vi "Actor Core.vi"(8 "error in":errorcluster, 11 "State in":refnum<class "Driver-Virtual.lvclass">) -> (0 "error out":errorcluster, 3 "Actor out":refnum<class "Actor.lvclass">)   [LabVIEW 2013, in "Virtual Systems.lvlib" / "Driver.lvlib" / "Driver-Virtual.lvclass"]
doc: "(<B>Filename</B>: Actor Framework.lvlib:Actor.lvclass:Actor Core.vi)\n\nThis override invokes Entry.vi on the initial state, prior to calling the parent Actor Core. Adding this behavior to Actor Core (instead of an override of Pre Launch Init.vi) allows the initial state to launch a nested actor as part of its entry behavior.\n\nReceives messages to the actor, reacts to them, and initiates any error handling that may shut the actor down.\n\nDescendant classes may override this VI to append parallel tasks for the actor to complete while it handles messages. Overrides use the Call Parent Method node."
uses:
  Driver-Virtual.lvclass
  Robot/Logical Systems/Driver/Driver-Logical/Driver.lvclass
  <vilib>/ActorFramework/Actor/Actor.lvclass
  Robot/Robot Actors/System Actor/System Actor Class/System Status.ctl
  Robot/Robot Actors/System Actor/System Actor Class/System Actor.lvclass
  Robot/Virtual Systems/XBox Controller/XBox Controller Class/Joystick.ctl
  Robot/Logical Systems/XBox Controller/XBox Controller Class/Xbox Controller.lvlib
  Robot/Logical Systems/XBox Controller/Xbox Controller.ctl
  Robot/Robot Actors/Command/Command Class/Command Status.ctl
  Robot/Robot Actors/Command/Command Class/Command.lvclass
  Robot/Robot Actors/Command/Command Class/Command States.ctl
  Robot/Robot Actors/Command Processor/Command Processor Class/Command Processor Status.ctl
  Robot/Robot Actors/Command Processor/Command Processor Class/Command Processor.lvclass
  Robot/Robot Actors/Command Processor/Command Processor Class/Command Processor States.ctl
panel:
  in  "Xbox Controller":T1 {"Right Joystick"."Right" min=-1.0 max=1.0 step=0.1 scale=-1.0..1.0; "Right Joystick"."Forward" min=-1.0 max=1.0 step=0.1 scale=-1.0..1.0; "Left Joystick"."Right" min=-1.0 max=1.0 step=0.1 scale=-1.0..1.0; "Left Joystick"."Forward" min=-1.0 max=1.0 step=0.1 scale=-1.0..1.0}
  in  "System Status":T3
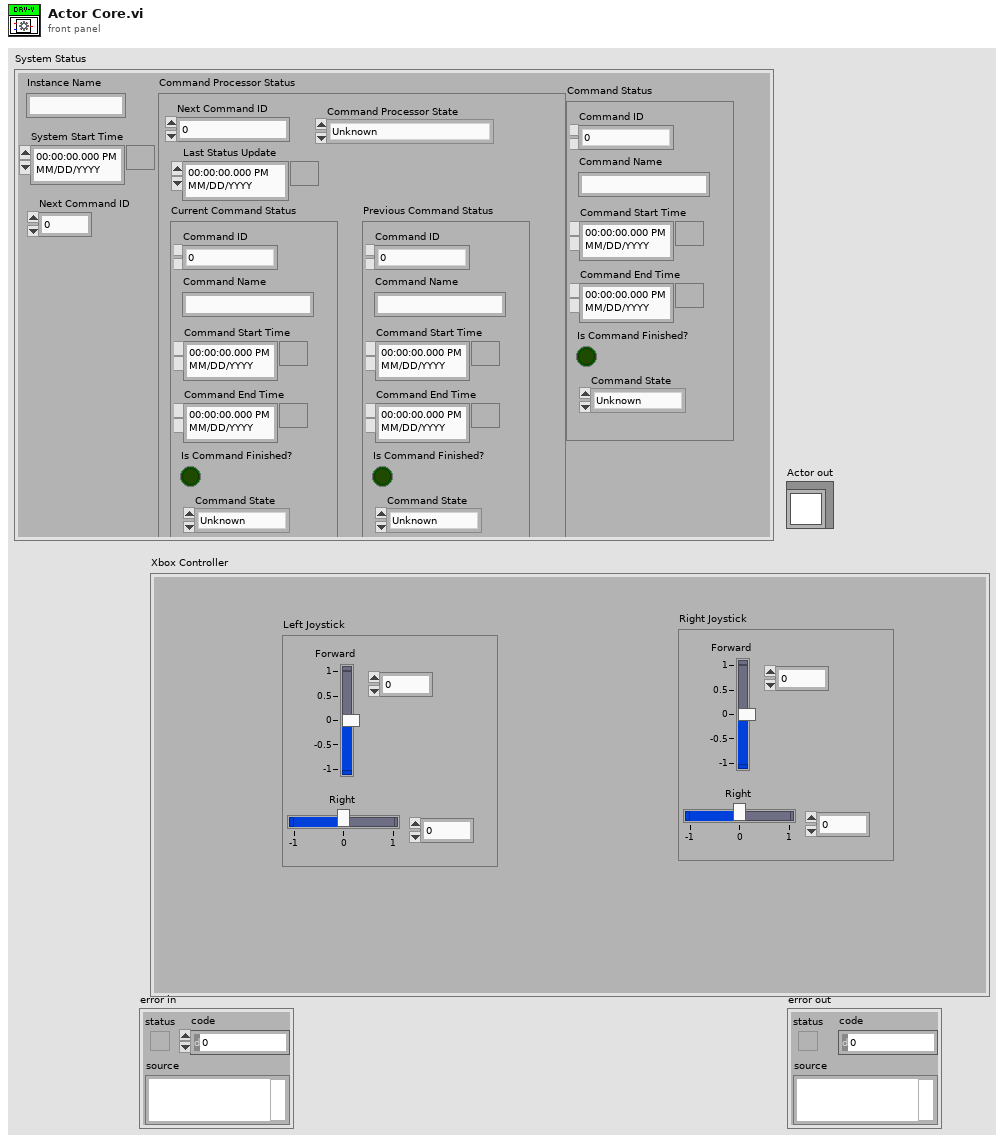
[diagram p1: front panel]
types:
  T1 = typedef "Logical Systems.lvlib/Xbox Controller.lvlib/Xbox Controller.ctl" = cluster{"Left Joystick":T2, "Right Joystick":T2}
  T2 = typedef "Logical Systems.lvlib/Xbox Controller.lvlib/Joystick.ctl" = cluster{"Forward":dbl, "Right":dbl}
  T3 = typedef "Robot Actors.lvlib/System Actor.lvlib/System Actor.lvclass/System Status.ctl" = cluster{"Instance Name":string, "Command Status":T4, "System Start Time":timestamp, "Next Command ID":dbl, "Command Processor Status":T6}
  T4 = typedef "Robot Actors.lvlib/Command.lvlib/Command.lvclass/Command Status.ctl" = cluster{"Command Name":string, "Command Start Time":timestamp, "Command End Time":timestamp, "Is Command Finished?":bool, "Command ID":dbl, "Command State":T5}
  T5 = typedef "Robot Actors.lvlib/Command.lvlib/Command.lvclass/Command States.ctl" = enum16{"Unknown", "Started", "Stopped", "Finished"}
  T6 = typedef "Robot Actors.lvlib/Command Processor.lvlib/Command Processor.lvclass/Command Processor Status.ctl" = cluster{"Next Command ID":dbl, "Current Command Status":T4, "Previous Command Status ":T4, "Command Processor State":T7, "Last Status Update":timestamp}
  T7 = typedef "Robot Actors.lvlib/Command Processor.lvlib/Command Processor.lvclass/Command Processor States.ctl" = enum16{"Unknown", "No Command", "Running Command"}
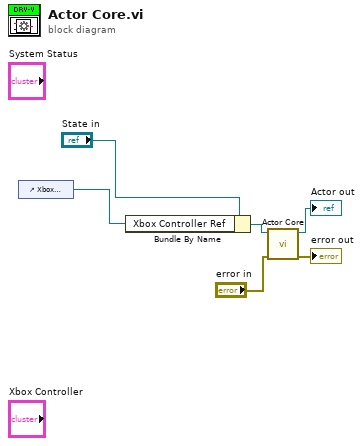
[diagram p0: block diagram]
diagram:
  n1 = control-ref of="Xbox Controller"() -> (w1:refnum<vi>)
  n2 = Bundle By Name(cluster="State in", "Xbox Controller Ref"=w1) -> (w2:refnum<class "Driver-Virtual.lvclass">)
  n3 = call-parent "Actor Core.vi"("error in"="error in", "State in"=w2) -> ("error out"=→"error out":errorcluster, "Actor out"=→"Actor out":refnum<class "Actor.lvclass">)  [unwired: 8 in]
